vi "9.生成模拟信号.vi"   [LabVIEW 2019]
uses:
  <vilib>/rvi/Emulation/niFpgaGetClockAttributes.vi
  <vilib>/rvi/Emulation/niFpgaSctlEmulationGetInTimedLoop.vi
  <vilib>/rvi/Emulation/niFpgaEmulationReportErrorSimple.vi
  <vilib>/rvi/eio/common/nirviEmuTemplateMethod_errors.vi
  <vilib>/rvi/Emulation/niFpgaCriticalErrorInLSC.vi
  <vilib>/rvi/FXPMathLib/FxpInterpret/XNode/nifxpmath_Interpret.xnode
  <vilib>/eio/EIONode/EIONode.xnode
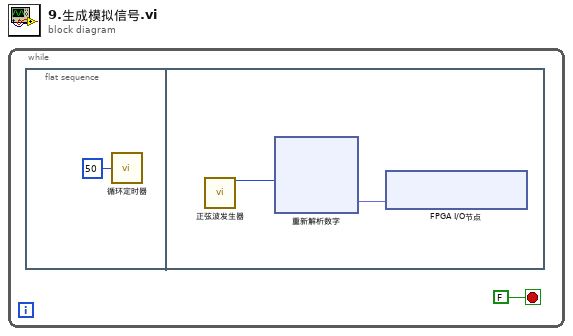
[diagram p0: block diagram]
diagram:
  n1 = while {
    stop <- FALSE stop-if-true
    n2 = flat-sequence {
      frame #0 {
        n3 = call "循环定时器"("Count(Ticks)"=u32 50) -> ()  [unwired: 1 out]
      }
      frame #1 {
        n4 = call "正弦波发生器"() -> ("sine out"=w4:i16)  [unwired: 15 in]
        n5 = xnode "重新解析数字"("x"=w4) -> ("y"=w3:fxp<+/-,16,4>)
        n6 = xnode "FPGA I/O节点"("ConnectorA/AO0"=w3) -> ()  [unwired: 1 in, 1 out]
      }
    }
  }
